vi "Core Actor - Close User Events.vi"(8 "error in (no error)":errorcluster, 11 "Interface_Class in":refnum<class "SW_Interface_Class.lvclass">) -> (0 "error out":errorcluster, 3 "Interface_Class out":refnum<class "SW_Interface_Class.lvclass">)   [LabVIEW 2023, in "SW_Interface_Actor.lvlib" / "SW_Interface_Class.lvclass"]
uses:
  SW_Interface_Class.lvclass
  Abstraction_Interface_Class/Abstraction_Interface_Class.lvclass
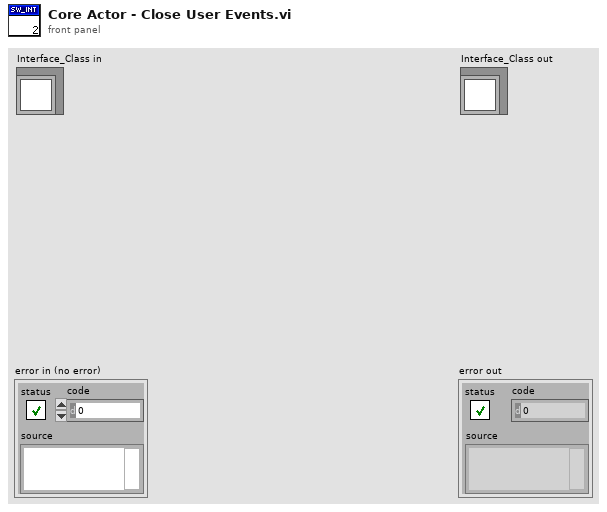
[diagram p1: front panel]
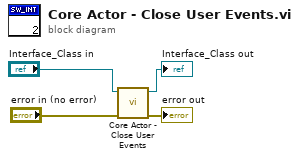
[diagram p0: block diagram]
diagram:
  n1 = call-parent "Core Actor - Close User Events.vi"("error in (no error)"="error in (no error)", "Interface_Class in"="Interface_Class in") -> ("error out"=→"error out":errorcluster, "Interface_Class out"=→"Interface_Class out":refnum<class "SW_Interface_Class.lvclass">)  [unwired: 8 in]
